vi "Deploy Model.vi"(7 "Remote Directory":string="models", 8 "Password":string, 9 "Username":string, 10 "Target IP Address":string, 11 "Local Model Path":path) -> (0 "error out":errorcluster, 3 "Remote File Path":string)   [LabVIEW 2020]
doc: "This VI will deploy a compiled model into <b>/home/lvuser/<Remote Directory></b> on the Linux-RT target specified by <b>Target IP Address</b>. If your target has permissions configured, you must provide the <b>Username</b> and <b>Password</b> for your target."
uses:
  <vilib>/WebDAVClient/NI_WebDAV.lvlib
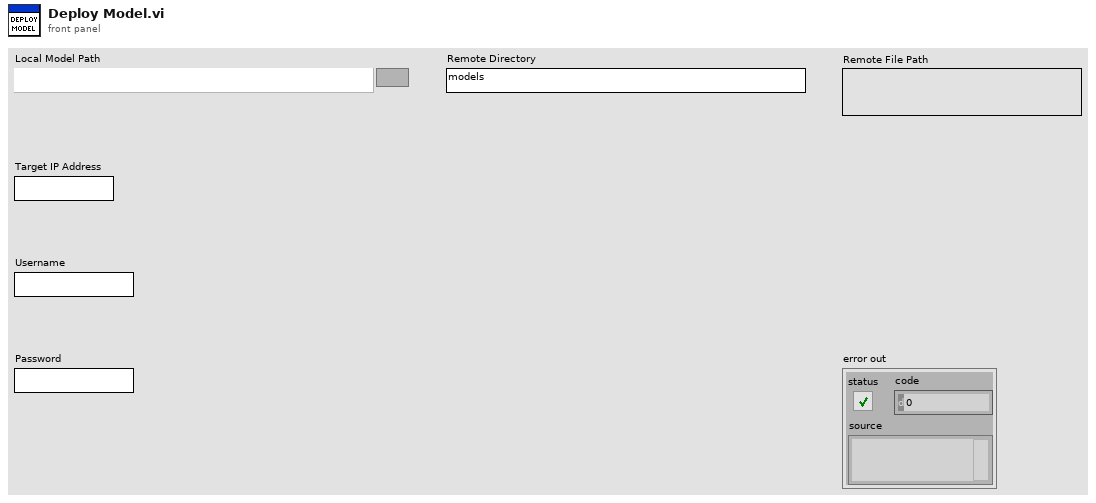
[diagram p1: front panel]
types:
  T1 = typedef "NI_WebDAV.lvlib/SessionHandle.ctl" = refnum<k1>
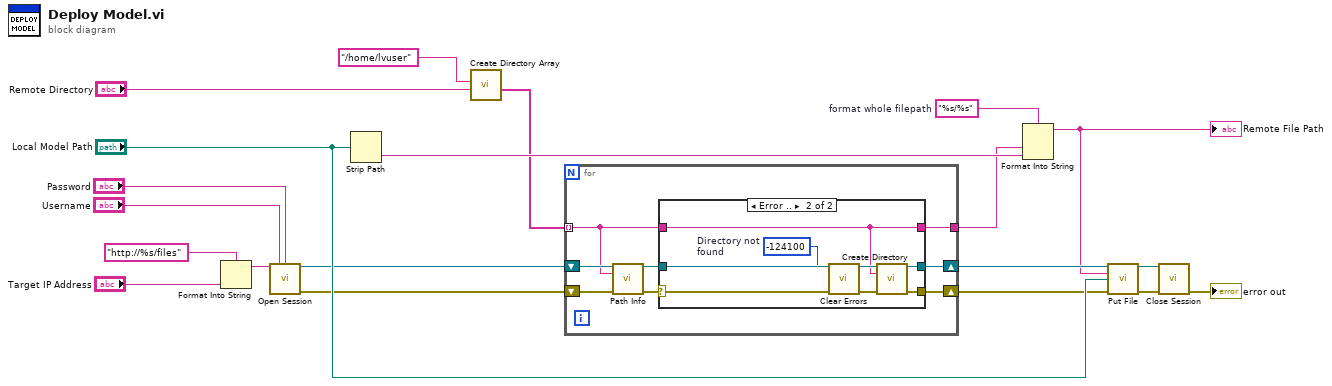
[diagram p0: block diagram]
diagram:
  w12 = "%s/%s"  # format whole filepath
  n1 = Format Into String(format string="http://%s/files" ("file uri"), "Target IP Address") -> (resulting string=w13:string)  [unwired: 2 in, 1 out]
  n2 = call <vilib>:"Open Session.vi"("host uri prefix"=w13, "username"="Username", "password"="Password") -> ("session handle out"=w5:T1, "error out"=w9:errorcluster)  [unwired: 11 in]
  n3 = Strip Path(path="Local Model Path") -> (name=w11:string)  [unwired: 1 out]
  n4 = call "Create Directory Array.vi"("Relative Path"="Remote Directory", "Root Folder"="/home/lvuser") -> ("Directory Array"=w1:string[])  [unwired: 9 in]
  n5 = for {
    shift-right: [w28] -> w15
    shift-left: w9 -> [w26]
    shift-right: [w27] -> w14
    shift-left: w5 -> [w23]
    tunnel: w1 -> [w21] mode=indexing
    tunnel: [w22] -> w4
    n6 = call <vilib>:"Path Info.vi"("session handle"=w23, "relative uri"=w21, "error in (no error)"=w26) -> ("session handle out"=w24:T1, "error out"=w25:errorcluster)  [unwired: 9 in, 2 out]
    n7 = case shown="Error .." w25 {
      selector: w25 -> [w30 w38]
      tunnel: [w30 w37] -> w28
      tunnel: w24 -> [w31 w36]
      tunnel: [w31 w35] -> w27
      tunnel: w21 -> [w29 w32]
      tunnel: [w29 w32] -> w22
      frame No Error {
      }
      frame Error {
        w33 = -124100  # Directory not found
        n8 = call <vilib>:"Clear Errors.vi"("error in (no error)"=w38, "specific error code to clear (0: all)"=w33) -> ("error out"=w34:errorcluster)  [unwired: 4 in, 1 out]
        n9 = call <vilib>:"Create Directory.vi"("session handle"=w36, "relative uri"=w32, "error in (no error)"=w34) -> ("session handle out"=w35:T1, "error out"=w37:errorcluster)  [unwired: 11 in]
      }
    }
  }
  n10 = Format Into String(format string=w12, w4, w11) -> (resulting string=w10:string)  [unwired: 2 in, 1 out]
  "Remote File Path" <- w10
  n11 = call <vilib>:"Put File.vi"("session handle"=w14, "relative uri"=w10, "local file path"="Local Model Path", "error in (no error)"=w15) -> ("session handle out"=w16:T1, "error out"=w17:errorcluster)  [unwired: 9 in, 1 out]
  n12 = call <vilib>:"Close Session.vi"("session handle"=w16, "error in (no error)"=w17) -> ("error out"=→"error out":errorcluster)  [unwired: 13 in]
